vi "Read Owner.vi"(9 "Generic in":refnum<class "Generic.lvclass">) -> (3 "Generic out":refnum<class "Generic.lvclass">, 4 "Owner":refnum<vi>)   [LabVIEW 2014, in "Generic.lvclass"]
uses:
  Generic.lvclass
  Generic.lvclass/Generic.ctl
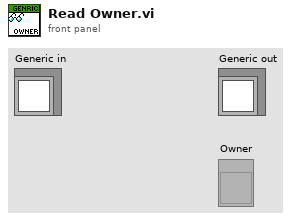
[diagram p1: front panel]
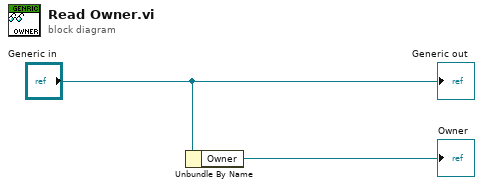
[diagram p0: block diagram]
diagram:
  n1 = Unbundle By Name("Generic in") -> ("Owner"=→"Owner":refnum<vi>)
  "Generic out" <- "Generic in"
